vi "DP-Show Comparison List.vi"(8 "error in (no error)":errorcluster, 10 "Listbox Ref":refnum<vi>, 11 "Comparison list":T1) -> (0 "error out":errorcluster)   [LabVIEW 2020]
uses:
  Typedefs/DP-Comparison List.ctl
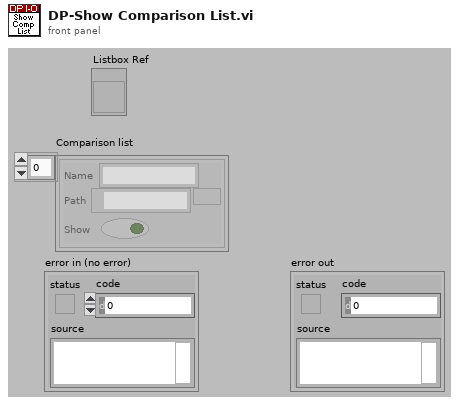
[diagram p1: front panel]
types:
  T1 = typedef "DP-Comparison List.ctl" = cluster{"Name":string, "Path":path, "Show":bool}[]
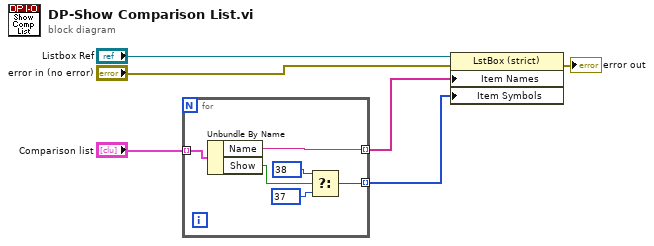
[diagram p0: block diagram]
diagram:
  n1 = for {
    tunnel: "Comparison list" -> [w12] mode=indexing
    tunnel: [w11] -> w5 mode=indexing
    tunnel: [w7] -> w4 mode=indexing
    n2 = Unbundle By Name(w12) -> ("Name"=w11:string, "Show"=w10:bool)
    n3 = Select(t=38, s=w10, f=37) -> (s? t:f=w7:i32)
  }
  n4 = property class="LstBox (strict)"(reference="Listbox Ref", error in="error in (no error)", "Item Names"=w5, "Item Symbols"=w4) -> (error out=→"error out":errorcluster)  [unwired: 1 out]
